vi "Get Socket Physical Name.vi"(8 "error In":errorcluster, 10 "ChannelType":string) -> (0 "error out":errorcluster, 2 "Physical Channel":tag[](array[tag]), 3 "Physical String":string[](array[string]))   [LabVIEW 2023, in "HardwareAbstractionLayer_LVOOP.lvlib" / "Teststand.lvclass"]
doc: "This VI Filter Physical Channel and Number Socket Running"
uses:
  Teststand.lvclass
  Database/Database.lvclass
panel:
  in  "Number Of DUT":i32
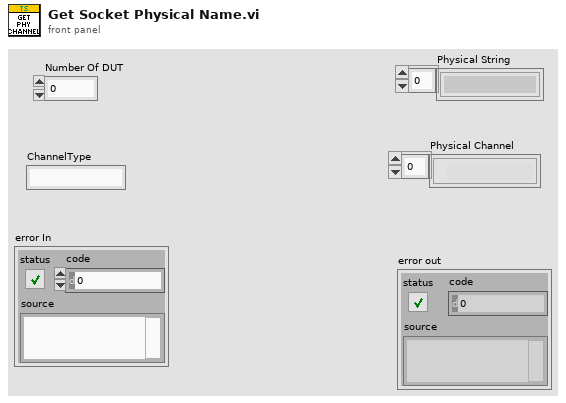
[diagram p1: front panel]
types:
  T1 = typedef "HardwareAbstractionLayer_LVOOP.lvlib/Teststand.lvclass/Teststand Status Control.ctl" = cluster{"Terminating or Aborting":bool, "Stop":bool, "Socket Count":i16, "Selected Sockets":i16[]}
  T2 = cluster{"table":string, "condition":string, "columns":string[]}
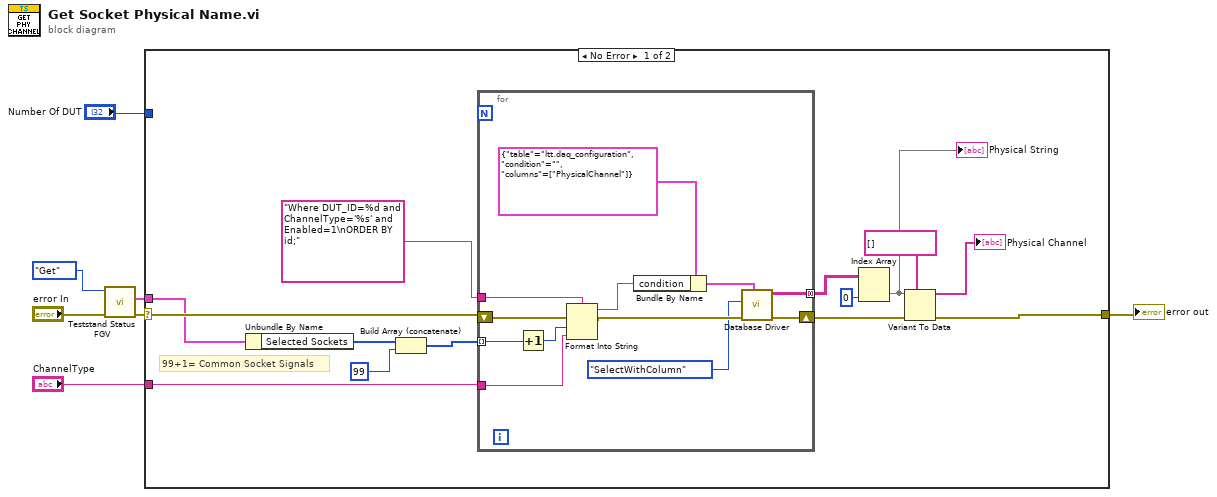
[diagram p0: block diagram]
diagram:
  n1 = call "Teststand Status FGV.vi"("error in"="error In", "Option"=enum16{"Set", "Get"}."Get") -> ("error out"=w3:errorcluster, "Teststand Status Out"=w2:T1)  [unwired: 8 in]
  n2 = case shown="No Error" w3 {
    selector: w3 -> [w15 w34]
    tunnel: "ChannelType" -> [w13 _]
    tunnel: [w12 w34] -> w6
    tunnel: w2 -> [w11 _]
    tunnel: "Number Of DUT" -> [_ _]
    frame No Error {
      # "99+1= Common Socket Signals"
      n3 = Unbundle By Name(w11) -> ("Selected Sockets"=w10:i16[])
      n4 = Build Array (concatenate)(w10, 99 ("Numeric")) -> (w9:i32[])
      n5 = for {
        tunnel: "Where DUT_ID=%d and ChannelType='%s' and Enabled=1\nORDER BY id;" -> [w33]
        shift-right: [w25] -> w21
        shift-left: w15 -> [w29]
        tunnel: [w24] -> w20 mode=concatenating
        tunnel: w13 -> [w28]
        tunnel: w9 -> [w22] mode=indexing
        n6 = Increment(x=w22) -> (x+1=w32:i32)
        n7 = Format Into String(format string=w33, error in=w29, w32, w28) -> (resulting string=w30:string, error out=w26:errorcluster)  [unwired: 1 in]
        n8 = Bundle By Name(cluster=T2 {"table"="ltt.daq_configuration", "condition"="", "columns"=["PhysicalChannel"]} ("SQLTableData"), "condition"=w30) -> (w27:T2)
        n9 = call "Database Driver.vi"("SQLTableData"=w27, "error in"=w26, "Select"=enum16{"SelectWithQuery", "SelectWithColumn"}."SelectWithColumn") -> ("error out"=w25:errorcluster, "data"=w24:string[][])  [unwired: 5 in, 2 out]
      }
      n10 = Index Array(array=w20, index (col)=0 ("disabled index (col)")) -> (element=w19:string[])  [unwired: 1 in]
      "Physical String" <- w19
      n11 = Variant To Data(error in=w21, type=tag[] [] ("AI.PhysicalChans"), Variant=w19) -> (data=→"Physical Channel":tag[], error out=w12:errorcluster)
    }
    frame Error {
    }
  }
  "error out" <- w6
